vi "FlexDDS-NG_USB_Example.vi"() -> ()   [LabVIEW 2010]
uses:
  <vilib>/Utility/xml.llb/Read From XML File(string).vi
  <vilib>/Utility/xml.llb/Write to XML File(string).vi
panel:
  in  "Interactive on/off":T1(ring)
  out "return count":u32=6435
  in  "Store data":enum32{"Save settings", "Don't save settings"}(tab)=enum."Don't save settings"
  in  "XML File Path WRITE":path=path "U:/Dokumente/Bachelorarbeit/Labview/FlexDDS-NG/conf/settings_s_curve_up_down.xml"
  in  "Data source":T2(tab)=enum."Generate data with function"
  in  "XML File Path READ":path=path "U:/Dokumente/Bachelorarbeit/Labview/FlexDDS-NG/conf/settings_4consecutive_falling.xml"
  in  "Select curve form":enum32{"S curve", "Exp curve"}(tab)
  in  "s curve parameters":cluster{"k":dbl}={"k"=10.0}
  in  "exp curve parameters":cluster{"k":dbl}={"k"=5.0}
  in  "parameters non-constant channel":T3={"Number of steps"=40, "time [ms]"=10000.0, "start frequency [Hz]"=80000000.0, "end frequency [Hz]"=82000000.0}
  in  "constant frequency":dbl=80000000.0 format="%#_13g"
  in  "Constant Channel":T4(ring)
  in  "CFR2 bits":T5={"Enable ASF from STP (F)"=FALSE, "Digital ramp enable (F)"=TRUE, "Digital ramp no-dwell high (F)"=FALSE, "Digital ramp no-dwell low (F)"=FALSE, "Matched latency enable (T)"=TRUE, "Parallel data port enable (F)"=FALSE}
  in  "CFR1 bits":T6={"RAM enable (F)"=FALSE, "Manual OSK external control (F)"=FALSE, "Inverse sinc filter enable (T)"=TRUE, "DDS sine (/cosine) output (F)"=FALSE, "Load LRR at I/O update (F)"=FALSE, "Autoclear digital ramp accumulator (F)"=TRUE, "Autoclear phase accumulator (F)"=FALSE, "Clear digital ramp accumulator (F)"=FALSE, "Clear phase accumulator (F)"=FALSE, "Load ARR at I/O update (F)"=FALSE, "OSK enable (F)"=FALSE, "Select Auto OSK (F)"=FALSE}
  in  "Trigger before sequence of sweeps":T7(ring)
  out "appended instruction string 2":string="dds reset\rdcp spi:CFR1=0x404000\rdcp spi:CFR2=0x80080\rdcp 0 spi:STP0=0x3FFF0000028F5C29\rdcp 1 spi:STP0=0x3FFF0000028F5C29\rdcp 0 spi:DRL=0x147C0118147BC1DB\rdcp 0 spi:DRSS=0xFFFFFFFF00000003\rdcp 0 spi:DRR=0x2D3E\rdcp 0 update:u-d\rdcp 0 update:+d\rdcp 1 spi:DRL=0x147AE148147AE148\rdcp 1 spi:DRSS=0xFFFFFFFF00000000\rdcp 1 spi:DRR=0xFFFF\rdcp 1 update:u-d\rdcp 1 update:+d\rdcp wait:1h:\rdcp wait::DROVER\rdcp 0 spi:DRL=0x147C51F1147C0118\rdcp 0 spi:DRSS=0xFFFFFFFF00000004\rdcp 0 spi:DRR=0x2F2F\rdcp 0 update:u-d\rdcp 0 update:+d\rdcp wait:1h:\rdcp wait::DROVER\rdcp 0 spi:DRL=0x147CB92D147C51F1\rdcp 0 spi:DRSS=0xFFFFFFFF00000017\rdcp 0 spi:DRR=0xD478\rdcp 0 update:u-d\rdcp 0 update:+d\rdcp wait:1h:\rdcp wait::DROVER\rdcp 0 spi:DRL=0x147D3CCC147CB92D\rdcp 0 spi:DRSS=0xFFFFFFFF00000009\rdcp 0 spi:DRR=0x4136\rdcp 0 update:u-d\rdcp 0 update:+d\rdcp wait:1h:\rdcp wait::DROVER\rdcp 0 spi:DRL=0x147DE446147D3CCC\rdcp 0 spi:DRSS=0xFFFFFFFF0000000D\rdcp 0 spi:DRR=0x4A07\rdcp 0 update:u-d\rdcp 0 update:+d\rdcp wait:1h:\rdcp wait::DROVER\rdcp 0 spi:DRL=0x147EB8D6147DE446\rdcp 0 spi:DRSS=0xFFFFFFFF0000002B\rdcp 0 spi:DRR=0xC0EC\rdcp 0 update:u-d\rdcp 0 update:+d\rdcp wait:1h:\rdcp wait::DROVER\rdcp 0 spi:DRL=0x147FC5C3147EB8D6\rdcp 0 spi:DRSS=0xFFFFFFFF00000006\rdcp 0 spi:DRR=0x1547\rdcp 0 update:u-d\rdcp 0 update:+d\rdcp wait:1h:\rdcp wait::DROVER\rdcp 0 spi:DRL=0x148118A1147FC5C3\rdcp 0 spi:DRSS=0xFFFFFFFF0000001C\rdcp 0 spi:DRR=0x4ECD\rdcp 0 update:u-d\rdcp 0 update:+d\rdcp wait:1h:\rdcp wait::DROVER\rdcp 0 spi:DRL=0x1482C174148118A1\rdcp 0 spi:DRSS=0xFFFFFFFF00000049\rdcp 0 spi:DRR=0xA3E0\rdcp 0 update:u-d\rdcp 0 update:+d\rdcp wait:1h:\rdcp wait::DROVER\rdcp 0 spi:DRL=0x1484D2A81482C174\rdcp 0 spi:DRSS=0xFFFFFFFF00000003\rdcp 0 spi:DRR=0x568\rdcp 0 update:u-d\rdcp 0 update:+d\rdcp wait:1h:\rdcp wait::DROVER\rdcp 0 spi:DRL=0x148760AD1484D2A8\rdcp 0 spi:DRSS=0xFFFFFFFF0000008C\rdcp 0 spi:DRR=0xCC25\rdcp 0 update:u-d\rdcp 0 update:+d\rdcp wait:1h:\rdcp wait::DROVER\rdcp 0 spi:DRL=0x148A8111148760AD\rdcp 0 spi:DRSS=0xFFFFFFFF00000049\rdcp 0 spi:DRR=0x56FB\rdcp 0 update:u-d\rdcp 0 update:+d\rdcp wait:1h:\rdcp wait::DROVER\rdcp 0 spi:DRL=0x148E48EB148A8111\rdcp 0 spi:DRSS=0xFFFFFFFF00000004\rdcp 0 spi:DRR=0x3F1\rdcp 0 update:u-d\rdcp 0 update:+d\rdcp wait:1h:\rdcp wait::DROVER\rdcp 0 spi:DRL=0x1492CA77148E48EB\rdcp 0 spi:DRSS=0xFFFFFFFF000000A0\rdcp 0 spi:DRR=0x8447\rdcp 0 update:u-d\rdcp 0 update:+d\rdcp wait:1h:\rdcp wait::DROVER\rdcp 0 spi:DRL=0x149811DB1492CA77\rdcp 0 spi:DRSS=0xFFFFFFFF000000D0\rdcp 0 spi:DRR=0x92C9\rdcp 0 update:u-d\rdcp 0 update:+d\rdcp wait:1h:\rdcp wait::DROVER\rdcp 0 spi:DRL=0x149E2175149811DB\rdcp 0 spi:DRSS=0xFFFFFFFF00000100\rdcp 0 spi:DRR=0x9D59\rdcp 0 update:u-d\rdcp 0 update:+d\rdcp wait:1h:\rdcp wait::DROVER\rdcp 0 spi:DRL=0x14A4EE42149E2175\rdcp 0 spi:DRSS=0xFFFFFFFF000000C7\rdcp 0 spi:DRR=0x6D05\rdcp 0 update:u-d\rdcp 0 update:+d\rdcp wait:1h:\rdcp wait::DROVER\rdcp 0 spi:DRL=0x14AC5D7114A4EE42\rdcp 0 spi:DRSS=0xFFFFFFFF00000019\rdcp 0 spi:DRR=0xC87\rdcp 0 update:u-d\rdcp 0 update:+d\rdcp wait:1h:\rdcp wait::DROVER\rdcp 0 spi:DRL=0x14B4443314AC5D71\rdcp 0 spi:DRSS=0xFFFFFFFF00000021\rdcp 0 spi:DRR=0xF8F\rdcp 0 update:u-d\rdcp 0 update:+d\rdcp wait:1h:\rdcp wait::DROVER\rdcp 0 spi:DRL=0x14BC6A7F14B44433\rdcp 0 spi:DRSS=0xFFFFFFFF0000014D\rdcp 0 spi:DRR=0x9838\rdcp 0 update:u-d\rdcp 0 update:+d\rdcp wait:1h:\rdcp wait::DROVER\rdcp 0 spi:DRL=0x14C490CB14BC6A7F\rdcp 0 spi:DRSS=0xFFFFFFFF0000014D\rdcp 0 spi:DRR=0x9838\rdcp 0 update:u-d\rdcp 0 update:+d\rdcp wait:1h:\rdcp wait::DROVER\rdcp 0 spi:DRL=0x14CC778D14C490CB\rdcp 0 spi:DRSS=0xFFFFFFFF00000021\rdcp 0 spi:DRR=0xF8F\rdcp 0 update:u-d\rdcp 0 update:+d\rdcp wait:1h:\rdcp wait::DROVER\rdcp 0 spi:DRL=0x14D3E6BC14CC778D\rdcp 0 spi:DRSS=0xFFFFFFFF00000019\rdcp 0 spi:DRR=0xC87\rdcp 0 update:u-d\rdcp 0 update:+d\rdcp wait:1h:\rdcp wait::DROVER\rdcp 0 spi:DRL=0x14DAB38914D3E6BC\rdcp 0 spi:DRSS=0xFFFFFFFF000000C7\rdcp 0 spi:DRR=0x6D05\rdcp 0 update:u-d\rdcp 0 update:+d\rdcp wait:1h:\rdcp wait::DROVER\rdcp 0 spi:DRL=0x14E0C32314DAB389\rdcp 0 spi:DRSS=0xFFFFFFFF00000100\rdcp 0 spi:DRR=0x9D59\rdcp 0 update:u-d\rdcp 0 update:+d\rdcp wait:1h:\rdcp wait::DROVER\rdcp 0 spi:DRL=0x14E60A8714E0C323\rdcp 0 spi:DRSS=0xFFFFFFFF000000D0\rdcp 0 spi:DRR=0x92C9\rdcp 0 update:u-d\rdcp 0 update:+d\rdcp wait:1h:\rdcp wait::DROVER\rdcp 0 spi:DRL=0x14EA8C1314E60A87\rdcp 0 spi:DRSS=0xFFFFFFFF000000A0\rdcp 0 spi:DRR=0x8447\rdcp 0 update:u-d\rdcp 0 update:+d\rdcp wait:1h:\rdcp wait::DROVER\rdcp 0 spi:DRL=0x14EE53ED14EA8C13\rdcp 0 spi:DRSS=0xFFFFFFFF00000004\rdcp 0 spi:DRR=0x3F1\rdcp 0 update:u-d\rdcp 0 update:+d\rdcp wait:1h:\rdcp wait::DROVER\rdcp 0 spi:DRL=0x14F1745114EE53ED\rdcp 0 spi:DRSS=0xFFFFFFFF00000049\rdcp 0 spi:DRR=0x56FB\rdcp 0 update:u-d\rdcp 0 update:+d\rdcp wait:1h:\rdcp wait::DROVER\rdcp 0 spi:DRL=0x14F4025514F17451\rdcp 0 spi:DRSS=0xFFFFFFFF0000008C\rdcp 0 spi:DRR=0xCC25\rdcp 0 update:u-d\rdcp 0 update:+d\rdcp wait:1h:\rdcp wait::DROVER\rdcp 0 spi:DRL=0x14F6138A14F40255\rdcp 0 spi:DRSS=0xFFFFFFFF00000003\rdcp 0 spi:DRR=0x568\rdcp 0 update:u-d\rdcp 0 update:+d\rdcp wait:1h:\rdcp wait::DROVER\rdcp 0 spi:DRL=0x14F7BC5D14F6138A\rdcp 0 spi:DRSS=0xFFFFFFFF00000049\rdcp 0 spi:DRR=0xA3E0\rdcp 0 update:u-d\rdcp 0 update:+d\rdcp wait:1h:\rdcp wait::DROVER\rdcp 0 spi:DRL=0x14F90F3B14F7BC5D\rdcp 0 spi:DRSS=0xFFFFFFFF0000001C\rdcp 0 spi:DRR=0x4ECD\rdcp 0 update:u-d\rdcp 0 update:+d\rdcp wait:1h:\rdcp wait::DROVER\rdcp 0 spi:DRL=0x14FA1C2814F90F3B\rdcp 0 spi:DRSS=0xFFFFFFFF00000006\rdcp 0 spi:DRR=0x1547\rdcp 0 update:u-d\rdcp 0 update:+d\rdcp wait:1h:\rdcp wait::DROVER\rdcp 0 spi:DRL=0x14FAF0B814FA1C28\rdcp 0 spi:DRSS=0xFFFFFFFF0000002B\rdcp 0 spi:DRR=0xC0EC\rdcp 0 update:u-d\rdcp 0 update:+d\rdcp wait:1h:\rdcp wait::DROVER\rdcp 0 spi:DRL=0x14FB983214FAF0B8\rdcp 0 spi:DRSS=0xFFFFFFFF0000000D\rdcp 0 spi:DRR=0x4A07\rdcp 0 update:u-d\rdcp 0 update:+d\rdcp wait:1h:\rdcp wait::DROVER\rdcp 0 spi:DRL=0x14FC1BD114FB9832\rdcp 0 spi:DRSS=0xFFFFFFFF00000009\rdcp 0 spi:DRR=0x4136\rdcp 0 update:u-d\rdcp 0 update:+d\rdcp wait:1h:\rdcp wait::DROVER\rdcp 0 spi:DRL=0x14FC830D14FC1BD1\rdcp 0 spi:DRSS=0xFFFFFFFF00000017\rdcp 0 spi:DRR=0xD478\rdcp 0 update:u-d\rdcp 0 update:+d\rdcp wait:1h:\rdcp wait::DROVER\rdcp 0 spi:DRL=0x14FCD3E614FC830D\rdcp 0 spi:DRSS=0xFFFFFFFF00000004\rdcp 0 spi:DRR=0x2F2F\rdcp 0 update:u-d\rdcp 0 update:+d\rdcp wait:1h:\rdcp wait::DROVER\rdcp 0 spi:DRL=0x14FD132314FCD3E6\rdcp 0 spi:DRSS=0xFFFFFFFF00000003\rdcp 0 spi:DRR=0x2D3E\rdcp 0 update:u-d\rdcp 0 update:+d\rdcp wait:1h:\rdcp wait::DROVER\rdcp 0 spi:DRL=0x14FD448E14FD1323\rdcp 0 spi:DRSS=0xFFFFFFFF00000002\rdcp 0 spi:DRR=0x2699\rdcp 0 update:u-d\rdcp 0 update:+d\rdcp wait:1h:\rdcp wait::DROVER\rdcp start\r"
  out "frequency-time plot":T8(graph)=[{[{"total time[ms]"=0.0, "f1 [Hz] CH0"=80013385.70184857}, {"total time[ms]"=250.0, "f1 [Hz] CH0"=80017154.97082743}, {"total time[ms]"=250.0, "f1 [Hz] CH0"=80017154.97082743}, {"total time[ms]"=500.0, "f1 [Hz] CH0"=80021973.8852612}, {"total time[ms]"=500.0, "f1 [Hz] CH0"=80021973.8852612}, {"total time[ms]"=750.0, "f1 [Hz] CH0"=80028127.2540865}, {"total time[ms]"=750.0, "f1 [Hz] CH0"=80028127.2540865}, {"total time[ms]"=1000.0, "f1 [Hz] CH0"=80035972.41992418}, {"total time[ms]"=1000.0, "f1 [Hz] CH0"=80035972.41992418}, {"total time[ms]"=1250.0, "f1 [Hz] CH0"=80045954.73982005}, {"total time[ms]"=1250.0, "f1 [Hz] CH0"=80045954.73982005}, {"total time[ms]"=1500.0, "f1 [Hz] CH0"=80058624.46150272}, {"total time[ms]"=1500.0, "f1 [Hz] CH0"=80058624.46150272}, {"total time[ms]"=1750.0, "f1 [Hz] CH0"=80074653.77468826}, {"total time[ms]"=1750.0, "f1 [Hz] CH0"=80074653.77468826}, {"total time[ms]"=2000.0, "f1 [Hz] CH0"=80094851.74635513}, {"total time[ms]"=2000.0, "f1 [Hz] CH0"=80094851.74635513}, {"total time[ms]"=2250.0, "f1 [Hz] CH0"=80120173.30034801}, {"total time[ms]"=2250.0, "f1 [Hz] CH0"=80120173.30034801}, {"total time[ms]"=2500.0, "f1 [Hz] CH0"=80151716.36004248}, {"total time[ms]"=2500.0, "f1 [Hz] CH0"=80151716.36004248}, {"total time[ms]"=2750.0, "f1 [Hz] CH0"=80190698.92979822}, {"total time[ms]"=2750.0, "f1 [Hz] CH0"=80190698.92979822}, {"total time[ms]"=3000.0, "f1 [Hz] CH0"=80238405.84404424}, {"total time[ms]"=3000.0, "f1 [Hz] CH0"=80238405.84404424}, {"total time[ms]"=3250.0, "f1 [Hz] CH0"=80296094.39606337}, {"total time[ms]"=3250.0, "f1 [Hz] CH0"=80296094.39606337}, {"total time[ms]"=3500.0, "f1 [Hz] CH0"=80364851.04761271}, {"total time[ms]"=3500.0, "f1 [Hz] CH0"=80364851.04761271}, {"total time[ms]"=3750.0, "f1 [Hz] CH0"=80445400.27765062}, {"total time[ms]"=3750.0, "f1 [Hz] CH0"=80445400.27765062}, {"total time[ms]"=4000.0, "f1 [Hz] CH0"=80537882.84273998}, {"total time[ms]"=4000.0, "f1 [Hz] CH0"=80537882.84273998}, {"total time[ms]"=4250.0, "f1 [Hz] CH0"=80641642.60164921}, {"total time[ms]"=4250.0, "f1 [Hz] CH0"=80641642.60164921}, {"total time[ms]"=4500.0, "f1 [Hz] CH0"=80755081.3375963}, {"total time[ms]"=4500.0, "f1 [Hz] CH0"=80755081.3375963}, {"total time[ms]"=4750.0, "f1 [Hz] CH0"=80875646.9982284}, {"total time[ms]"=4750.0, "f1 [Hz] CH0"=80875646.9982284}, {"total time[ms]"=5000.0, "f1 [Hz] CH0"=81000000.0}, {"total time[ms]"=5000.0, "f1 [Hz] CH0"=81000000.0}, {"total time[ms]"=5250.0, "f1 [Hz] CH0"=81124353.0017716}, {"total time[ms]"=5250.0, "f1 [Hz] CH0"=81124353.0017716}, {"total time[ms]"=5500.0, "f1 [Hz] CH0"=81244918.6624037}, {"total time[ms]"=5500.0, "f1 [Hz] CH0"=81244918.6624037}, {"total time[ms]"=5750.0, "f1 [Hz] CH0"=81358357.39835079}, {"total time[ms]"=5750.0, "f1 [Hz] CH0"=81358357.39835079}, {"total time[ms]"=6000.0, "f1 [Hz] CH0"=81462117.15726002}, {"total time[ms]"=6000.0, "f1 [Hz] CH0"=81462117.15726002}, {"total time[ms]"=6250.0, "f1 [Hz] CH0"=81554599.72234938}, {"total time[ms]"=6250.0, "f1 [Hz] CH0"=81554599.72234938}, {"total time[ms]"=6500.0, "f1 [Hz] CH0"=81635148.95238729}, {"total time[ms]"=6500.0, "f1 [Hz] CH0"=81635148.95238729}, {"total time[ms]"=6750.0, "f1 [Hz] CH0"=81703905.60393663}, {"total time[ms]"=6750.0, "f1 [Hz] CH0"=81703905.60393663}, {"total time[ms]"=7000.0, "f1 [Hz] CH0"=81761594.15595576}, {"total time[ms]"=7000.0, "f1 [Hz] CH0"=81761594.15595576}, {"total time[ms]"=7250.0, "f1 [Hz] CH0"=81809301.07020178}, {"total time[ms]"=7250.0, "f1 [Hz] CH0"=81809301.07020178}, {"total time[ms]"=7500.0, "f1 [Hz] CH0"=81848283.63995752}, {"total time[ms]"=7500.0, "f1 [Hz] CH0"=81848283.63995752}, {"total time[ms]"=7750.0, "f1 [Hz] CH0"=81879826.69965199}, {"total time[ms]"=7750.0, "f1 [Hz] CH0"=81879826.69965199}, {"total time[ms]"=8000.0, "f1 [Hz] CH0"=81905148.25364487}, {"total time[ms]"=8000.0, "f1 [Hz] CH0"=81905148.25364487}, {"total time[ms]"=8250.0, "f1 [Hz] CH0"=81925346.22531174}, {"total time[ms]"=8250.0, "f1 [Hz] CH0"=81925346.22531174}, {"total time[ms]"=8500.0, "f1 [Hz] CH0"=81941375.53849728}, {"total time[ms]"=8500.0, "f1 [Hz] CH0"=81941375.53849728}, {"total time[ms]"=8750.0, "f1 [Hz] CH0"=81954045.26017995}, {"total time[ms]"=8750.0, "f1 [Hz] CH0"=81954045.26017995}, {"total time[ms]"=9000.0, "f1 [Hz] CH0"=81964027.58007582}, {"total time[ms]"=9000.0, "f1 [Hz] CH0"=81964027.58007582}, {"total time[ms]"=9250.0, "f1 [Hz] CH0"=81971872.7459135}, {"total time[ms]"=9250.0, "f1 [Hz] CH0"=81971872.7459135}, {"total time[ms]"=9500.0, "f1 [Hz] CH0"=81978026.1147388}, {"total time[ms]"=9500.0, "f1 [Hz] CH0"=81978026.1147388}, {"total time[ms]"=9750.0, "f1 [Hz] CH0"=81982845.02917257}, {"total time[ms]"=9750.0, "f1 [Hz] CH0"=81982845.02917257}, {"total time[ms]"=10000.0, "f1 [Hz] CH0"=81986614.29815143}, {"total time[ms]"=10000.0, "f1 [Hz] CH0"=81986614.29815143}, {"total time[ms]"=10250.0, "f1 [Hz] CH0"=81989559.74861288}]}, {[{"total time[ms]"=0.0, "f1 [Hz] CH0"=80000000.0}, {"total time[ms]"=250.0, "f1 [Hz] CH0"=80000000.0}, {"total time[ms]"=250.0, "f1 [Hz] CH0"=80000000.0}, {"total time[ms]"=500.0, "f1 [Hz] CH0"=80000000.0}, {"total time[ms]"=500.0, "f1 [Hz] CH0"=80000000.0}, {"total time[ms]"=750.0, "f1 [Hz] CH0"=80000000.0}, {"total time[ms]"=750.0, "f1 [Hz] CH0"=80000000.0}, {"total time[ms]"=1000.0, "f1 [Hz] CH0"=80000000.0}, {"total time[ms]"=1000.0, "f1 [Hz] CH0"=80000000.0}, {"total time[ms]"=1250.0, "f1 [Hz] CH0"=80000000.0}, {"total time[ms]"=1250.0, "f1 [Hz] CH0"=80000000.0}, {"total time[ms]"=1500.0, "f1 [Hz] CH0"=80000000.0}, {"total time[ms]"=1500.0, "f1 [Hz] CH0"=80000000.0}, {"total time[ms]"=1750.0, "f1 [Hz] CH0"=80000000.0}, {"total time[ms]"=1750.0, "f1 [Hz] CH0"=80000000.0}, {"total time[ms]"=2000.0, "f1 [Hz] CH0"=80000000.0}, {"total time[ms]"=2000.0, "f1 [Hz] CH0"=80000000.0}, {"total time[ms]"=2250.0, "f1 [Hz] CH0"=80000000.0}, {"total time[ms]"=2250.0, "f1 [Hz] CH0"=80000000.0}, {"total time[ms]"=2500.0, "f1 [Hz] CH0"=80000000.0}, {"total time[ms]"=2500.0, "f1 [Hz] CH0"=80000000.0}, {"total time[ms]"=2750.0, "f1 [Hz] CH0"=80000000.0}, {"total time[ms]"=2750.0, "f1 [Hz] CH0"=80000000.0}, {"total time[ms]"=3000.0, "f1 [Hz] CH0"=80000000.0}, {"total time[ms]"=3000.0, "f1 [Hz] CH0"=80000000.0}, {"total time[ms]"=3250.0, "f1 [Hz] CH0"=80000000.0}, {"total time[ms]"=3250.0, "f1 [Hz] CH0"=80000000.0}, {"total time[ms]"=3500.0, "f1 [Hz] CH0"=80000000.0}, {"total time[ms]"=3500.0, "f1 [Hz] CH0"=80000000.0}, {"total time[ms]"=3750.0, "f1 [Hz] CH0"=80000000.0}, {"total time[ms]"=3750.0, "f1 [Hz] CH0"=80000000.0}, {"total time[ms]"=4000.0, "f1 [Hz] CH0"=80000000.0}, {"total time[ms]"=4000.0, "f1 [Hz] CH0"=80000000.0}, {"total time[ms]"=4250.0, "f1 [Hz] CH0"=80000000.0}, {"total time[ms]"=4250.0, "f1 [Hz] CH0"=80000000.0}, {"total time[ms]"=4500.0, "f1 [Hz] CH0"=80000000.0}, {"total time[ms]"=4500.0, "f1 [Hz] CH0"=80000000.0}, {"total time[ms]"=4750.0, "f1 [Hz] CH0"=80000000.0}, {"total time[ms]"=4750.0, "f1 [Hz] CH0"=80000000.0}, {"total time[ms]"=5000.0, "f1 [Hz] CH0"=80000000.0}, {"total time[ms]"=5000.0, "f1 [Hz] CH0"=80000000.0}, {"total time[ms]"=5250.0, "f1 [Hz] CH0"=80000000.0}, {"total time[ms]"=5250.0, "f1 [Hz] CH0"=80000000.0}, {"total time[ms]"=5500.0, "f1 [Hz] CH0"=80000000.0}, {"total time[ms]"=5500.0, "f1 [Hz] CH0"=80000000.0}, {"total time[ms]"=5750.0, "f1 [Hz] CH0"=80000000.0}, {"total time[ms]"=5750.0, "f1 [Hz] CH0"=80000000.0}, {"total time[ms]"=6000.0, "f1 [Hz] CH0"=80000000.0}, {"total time[ms]"=6000.0, "f1 [Hz] CH0"=80000000.0}, {"total time[ms]"=6250.0, "f1 [Hz] CH0"=80000000.0}, {"total time[ms]"=6250.0, "f1 [Hz] CH0"=80000000.0}, {"total time[ms]"=6500.0, "f1 [Hz] CH0"=80000000.0}, {"total time[ms]"=6500.0, "f1 [Hz] CH0"=80000000.0}, {"total time[ms]"=6750.0, "f1 [Hz] CH0"=80000000.0}, {"total time[ms]"=6750.0, "f1 [Hz] CH0"=80000000.0}, {"total time[ms]"=7000.0, "f1 [Hz] CH0"=80000000.0}, {"total time[ms]"=7000.0, "f1 [Hz] CH0"=80000000.0}, {"total time[ms]"=7250.0, "f1 [Hz] CH0"=80000000.0}, {"total time[ms]"=7250.0, "f1 [Hz] CH0"=80000000.0}, {"total time[ms]"=7500.0, "f1 [Hz] CH0"=80000000.0}, {"total time[ms]"=7500.0, "f1 [Hz] CH0"=80000000.0}, {"total time[ms]"=7750.0, "f1 [Hz] CH0"=80000000.0}, {"total time[ms]"=7750.0, "f1 [Hz] CH0"=80000000.0}, {"total time[ms]"=8000.0, "f1 [Hz] CH0"=80000000.0}, {"total time[ms]"=8000.0, "f1 [Hz] CH0"=80000000.0}, {"total time[ms]"=8250.0, "f1 [Hz] CH0"=80000000.0}, {"total time[ms]"=8250.0, "f1 [Hz] CH0"=80000000.0}, {"total time[ms]"=8500.0, "f1 [Hz] CH0"=80000000.0}, {"total time[ms]"=8500.0, "f1 [Hz] CH0"=80000000.0}, {"total time[ms]"=8750.0, "f1 [Hz] CH0"=80000000.0}, {"total time[ms]"=8750.0, "f1 [Hz] CH0"=80000000.0}, {"total time[ms]"=9000.0, "f1 [Hz] CH0"=80000000.0}, {"total time[ms]"=9000.0, "f1 [Hz] CH0"=80000000.0}, {"total time[ms]"=9250.0, "f1 [Hz] CH0"=80000000.0}, {"total time[ms]"=9250.0, "f1 [Hz] CH0"=80000000.0}, {"total time[ms]"=9500.0, "f1 [Hz] CH0"=80000000.0}, {"total time[ms]"=9500.0, "f1 [Hz] CH0"=80000000.0}, {"total time[ms]"=9750.0, "f1 [Hz] CH0"=80000000.0}, {"total time[ms]"=9750.0, "f1 [Hz] CH0"=80000000.0}, {"total time[ms]"=10000.0, "f1 [Hz] CH0"=80000000.0}, {"total time[ms]"=10000.0, "f1 [Hz] CH0"=80000000.0}, {"total time[ms]"=10250.0, "f1 [Hz] CH0"=80000000.0}]}]
  in  "Control Elements Array":T9(array[cluster])=[{"STEP"=0, "time[ms]"=250.0, "time tolerance[us]"=0.01, "CH0"=TRUE, "rel. amplitude CH0"=1.0, "phase [°] CH0"=0.0, "f0 [Hz] CH0"=80013385.70184857, "f1 [Hz] CH0"=80017154.97082743, "CH1"=TRUE, "rel. amplitude CH1"=1.0, "phase [°] CH1"=0.0, "f0 [Hz] CH1"=80000000.0, "f1 [Hz] CH1"=80000000.0}, {"STEP"=0, "time[ms]"=250.0, "time tolerance[us]"=0.01, "CH0"=TRUE, "rel. amplitude CH0"=1.0, "phase [°] CH0"=0.0, "f0 [Hz] CH0"=80017154.97082743, "f1 [Hz] CH0"=80021973.8852612, "CH1"=FALSE, "rel. amplitude CH1"=1.0, "phase [°] CH1"=0.0, "f0 [Hz] CH1"=80000000.0, "f1 [Hz] CH1"=80000000.0}, {"STEP"=0, "time[ms]"=250.0, "time tolerance[us]"=0.01, "CH0"=TRUE, "rel. amplitude CH0"=1.0, "phase [°] CH0"=0.0, "f0 [Hz] CH0"=80021973.8852612, "f1 [Hz] CH0"=80028127.2540865, "CH1"=FALSE, "rel. amplitude CH1"=1.0, "phase [°] CH1"=0.0, "f0 [Hz] CH1"=80000000.0, "f1 [Hz] CH1"=80000000.0}, {"STEP"=0, "time[ms]"=250.0, "time tolerance[us]"=0.01, "CH0"=TRUE, "rel. amplitude CH0"=1.0, "phase [°] CH0"=0.0, "f0 [Hz] CH0"=80028127.2540865, "f1 [Hz] CH0"=80035972.41992418, "CH1"=FALSE, "rel. amplitude CH1"=1.0, "phase [°] CH1"=0.0, "f0 [Hz] CH1"=80000000.0, "f1 [Hz] CH1"=80000000.0}, {"STEP"=0, "time[ms]"=250.0, "time tolerance[us]"=0.01, "CH0"=TRUE, "rel. amplitude CH0"=1.0, "phase [°] CH0"=0.0, "f0 [Hz] CH0"=80035972.41992418, "f1 [Hz] CH0"=80045954.73982005, "CH1"=FALSE, "rel. amplitude CH1"=1.0, "phase [°] CH1"=0.0, "f0 [Hz] CH1"=80000000.0, "f1 [Hz] CH1"=80000000.0}, {"STEP"=0, "time[ms]"=250.0, "time tolerance[us]"=0.01, "CH0"=TRUE, "rel. amplitude CH0"=1.0, "phase [°] CH0"=0.0, "f0 [Hz] CH0"=80045954.73982005, "f1 [Hz] CH0"=80058624.46150272, "CH1"=FALSE, "rel. amplitude CH1"=1.0, "phase [°] CH1"=0.0, "f0 [Hz] CH1"=80000000.0, "f1 [Hz] CH1"=80000000.0}, {"STEP"=0, "time[ms]"=250.0, "time tolerance[us]"=0.01, "CH0"=TRUE, "rel. amplitude CH0"=1.0, "phase [°] CH0"=0.0, "f0 [Hz] CH0"=80058624.46150272, "f1 [Hz] CH0"=80074653.77468826, "CH1"=FALSE, "rel. amplitude CH1"=1.0, "phase [°] CH1"=0.0, "f0 [Hz] CH1"=80000000.0, "f1 [Hz] CH1"=80000000.0}, {"STEP"=0, "time[ms]"=250.0, "time tolerance[us]"=0.01, "CH0"=TRUE, "rel. amplitude CH0"=1.0, "phase [°] CH0"=0.0, "f0 [Hz] CH0"=80074653.77468826, "f1 [Hz] CH0"=80094851.74635513, "CH1"=FALSE, "rel. amplitude CH1"=1.0, "phase [°] CH1"=0.0, "f0 [Hz] CH1"=80000000.0, "f1 [Hz] CH1"=80000000.0}, {"STEP"=0, "time[ms]"=250.0, "time tolerance[us]"=0.01, "CH0"=TRUE, "rel. amplitude CH0"=1.0, "phase [°] CH0"=0.0, "f0 [Hz] CH0"=80094851.74635513, "f1 [Hz] CH0"=80120173.30034801, "CH1"=FALSE, "rel. amplitude CH1"=1.0, "phase [°] CH1"=0.0, "f0 [Hz] CH1"=80000000.0, "f1 [Hz] CH1"=80000000.0}, {"STEP"=0, "time[ms]"=250.0, "time tolerance[us]"=0.01, "CH0"=TRUE, "rel. amplitude CH0"=1.0, "phase [°] CH0"=0.0, "f0 [Hz] CH0"=80120173.30034801, "f1 [Hz] CH0"=80151716.36004248, "CH1"=FALSE, "rel. amplitude CH1"=1.0, "phase [°] CH1"=0.0, "f0 [Hz] CH1"=80000000.0, "f1 [Hz] CH1"=80000000.0}, {"STEP"=0, "time[ms]"=250.0, "time tolerance[us]"=0.01, "CH0"=TRUE, "rel. amplitude CH0"=1.0, "phase [°] CH0"=0.0, "f0 [Hz] CH0"=80151716.36004248, "f1 [Hz] CH0"=80190698.92979822, "CH1"=FALSE, "rel. amplitude CH1"=1.0, "phase [°] CH1"=0.0, "f0 [Hz] CH1"=80000000.0, "f1 [Hz] CH1"=80000000.0}, {"STEP"=0, "time[ms]"=250.0, "time tolerance[us]"=0.01, "CH0"=TRUE, "rel. amplitude CH0"=1.0, "phase [°] CH0"=0.0, "f0 [Hz] CH0"=80190698.92979822, "f1 [Hz] CH0"=80238405.84404424, "CH1"=FALSE, "rel. amplitude CH1"=1.0, "phase [°] CH1"=0.0, "f0 [Hz] CH1"=80000000.0, "f1 [Hz] CH1"=80000000.0}, {"STEP"=0, "time[ms]"=250.0, "time tolerance[us]"=0.01, "CH0"=TRUE, "rel. amplitude CH0"=1.0, "phase [°] CH0"=0.0, "f0 [Hz] CH0"=80238405.84404424, "f1 [Hz] CH0"=80296094.39606337, "CH1"=FALSE, "rel. amplitude CH1"=1.0, "phase [°] CH1"=0.0, "f0 [Hz] CH1"=80000000.0, "f1 [Hz] CH1"=80000000.0}, {"STEP"=0, "time[ms]"=250.0, "time tolerance[us]"=0.01, "CH0"=TRUE, "rel. amplitude CH0"=1.0, "phase [°] CH0"=0.0, "f0 [Hz] CH0"=80296094.39606337, "f1 [Hz] CH0"=80364851.04761271, "CH1"=FALSE, "rel. amplitude CH1"=1.0, "phase [°] CH1"=0.0, "f0 [Hz] CH1"=80000000.0, "f1 [Hz] CH1"=80000000.0}, {"STEP"=0, "time[ms]"=250.0, "time tolerance[us]"=0.01, "CH0"=TRUE, "rel. amplitude CH0"=1.0, "phase [°] CH0"=0.0, "f0 [Hz] CH0"=80364851.04761271, "f1 [Hz] CH0"=80445400.27765062, "CH1"=FALSE, "rel. amplitude CH1"=1.0, "phase [°] CH1"=0.0, "f0 [Hz] CH1"=80000000.0, "f1 [Hz] CH1"=80000000.0}, {"STEP"=0, "time[ms]"=250.0, "time tolerance[us]"=0.01, "CH0"=TRUE, "rel. amplitude CH0"=1.0, "phase [°] CH0"=0.0, "f0 [Hz] CH0"=80445400.27765062, "f1 [Hz] CH0"=80537882.84273998, "CH1"=FALSE, "rel. amplitude CH1"=1.0, "phase [°] CH1"=0.0, "f0 [Hz] CH1"=80000000.0, "f1 [Hz] CH1"=80000000.0}, {"STEP"=0, "time[ms]"=250.0, "time tolerance[us]"=0.01, "CH0"=TRUE, "rel. amplitude CH0"=1.0, "phase [°] CH0"=0.0, "f0 [Hz] CH0"=80537882.84273998, "f1 [Hz] CH0"=80641642.60164921, "CH1"=FALSE, "rel. amplitude CH1"=1.0, "phase [°] CH1"=0.0, "f0 [Hz] CH1"=80000000.0, "f1 [Hz] CH1"=80000000.0}, {"STEP"=0, "time[ms]"=250.0, "time tolerance[us]"=0.01, "CH0"=TRUE, "rel. amplitude CH0"=1.0, "phase [°] CH0"=0.0, "f0 [Hz] CH0"=80641642.60164921, "f1 [Hz] CH0"=80755081.3375963, "CH1"=FALSE, "rel. amplitude CH1"=1.0, "phase [°] CH1"=0.0, "f0 [Hz] CH1"=80000000.0, "f1 [Hz] CH1"=80000000.0}, {"STEP"=0, "time[ms]"=250.0, "time tolerance[us]"=0.01, "CH0"=TRUE, "rel. amplitude CH0"=1.0, "phase [°] CH0"=0.0, "f0 [Hz] CH0"=80755081.3375963, "f1 [Hz] CH0"=80875646.9982284, "CH1"=FALSE, "rel. amplitude CH1"=1.0, "phase [°] CH1"=0.0, "f0 [Hz] CH1"=80000000.0, "f1 [Hz] CH1"=80000000.0}, {"STEP"=0, "time[ms]"=250.0, "time tolerance[us]"=0.01, "CH0"=TRUE, "rel. amplitude CH0"=1.0, "phase [°] CH0"=0.0, "f0 [Hz] CH0"=80875646.9982284, "f1 [Hz] CH0"=81000000.0, "CH1"=FALSE, "rel. amplitude CH1"=1.0, "phase [°] CH1"=0.0, "f0 [Hz] CH1"=80000000.0, "f1 [Hz] CH1"=80000000.0}, {"STEP"=0, "time[ms]"=250.0, "time tolerance[us]"=0.01, "CH0"=TRUE, "rel. amplitude CH0"=1.0, "phase [°] CH0"=0.0, "f0 [Hz] CH0"=81000000.0, "f1 [Hz] CH0"=81124353.0017716, "CH1"=FALSE, "rel. amplitude CH1"=1.0, "phase [°] CH1"=0.0, "f0 [Hz] CH1"=80000000.0, "f1 [Hz] CH1"=80000000.0}, {"STEP"=0, "time[ms]"=250.0, "time tolerance[us]"=0.01, "CH0"=TRUE, "rel. amplitude CH0"=1.0, "phase [°] CH0"=0.0, "f0 [Hz] CH0"=81124353.0017716, "f1 [Hz] CH0"=81244918.6624037, "CH1"=FALSE, "rel. amplitude CH1"=1.0, "phase [°] CH1"=0.0, "f0 [Hz] CH1"=80000000.0, "f1 [Hz] CH1"=80000000.0}, {"STEP"=0, "time[ms]"=250.0, "time tolerance[us]"=0.01, "CH0"=TRUE, "rel. amplitude CH0"=1.0, "phase [°] CH0"=0.0, "f0 [Hz] CH0"=81244918.6624037, "f1 [Hz] CH0"=81358357.39835079, "CH1"=FALSE, "rel. amplitude CH1"=1.0, "phase [°] CH1"=0.0, "f0 [Hz] CH1"=80000000.0, "f1 [Hz] CH1"=80000000.0}, {"STEP"=0, "time[ms]"=250.0, "time tolerance[us]"=0.01, "CH0"=TRUE, "rel. amplitude CH0"=1.0, "phase [°] CH0"=0.0, "f0 [Hz] CH0"=81358357.39835079, "f1 [Hz] CH0"=81462117.15726002, "CH1"=FALSE, "rel. amplitude CH1"=1.0, "phase [°] CH1"=0.0, "f0 [Hz] CH1"=80000000.0, "f1 [Hz] CH1"=80000000.0}, {"STEP"=0, "time[ms]"=250.0, "time tolerance[us]"=0.01, "CH0"=TRUE, "rel. amplitude CH0"=1.0, "phase [°] CH0"=0.0, "f0 [Hz] CH0"=81462117.15726002, "f1 [Hz] CH0"=81554599.72234938, "CH1"=FALSE, "rel. amplitude CH1"=1.0, "phase [°] CH1"=0.0, "f0 [Hz] CH1"=80000000.0, "f1 [Hz] CH1"=80000000.0}, {"STEP"=0, "time[ms]"=250.0, "time tolerance[us]"=0.01, "CH0"=TRUE, "rel. amplitude CH0"=1.0, "phase [°] CH0"=0.0, "f0 [Hz] CH0"=81554599.72234938, "f1 [Hz] CH0"=81635148.95238729, "CH1"=FALSE, "rel. amplitude CH1"=1.0, "phase [°] CH1"=0.0, "f0 [Hz] CH1"=80000000.0, "f1 [Hz] CH1"=80000000.0}, {"STEP"=0, "time[ms]"=250.0, "time tolerance[us]"=0.01, "CH0"=TRUE, "rel. amplitude CH0"=1.0, "phase [°] CH0"=0.0, "f0 [Hz] CH0"=81635148.95238729, "f1 [Hz] CH0"=81703905.60393663, "CH1"=FALSE, "rel. amplitude CH1"=1.0, "phase [°] CH1"=0.0, "f0 [Hz] CH1"=80000000.0, "f1 [Hz] CH1"=80000000.0}, {"STEP"=0, "time[ms]"=250.0, "time tolerance[us]"=0.01, "CH0"=TRUE, "rel. amplitude CH0"=1.0, "phase [°] CH0"=0.0, "f0 [Hz] CH0"=81703905.60393663, "f1 [Hz] CH0"=81761594.15595576, "CH1"=FALSE, "rel. amplitude CH1"=1.0, "phase [°] CH1"=0.0, "f0 [Hz] CH1"=80000000.0, "f1 [Hz] CH1"=80000000.0}, {"STEP"=0, "time[ms]"=250.0, "time tolerance[us]"=0.01, "CH0"=TRUE, "rel. amplitude CH0"=1.0, "phase [°] CH0"=0.0, "f0 [Hz] CH0"=81761594.15595576, "f1 [Hz] CH0"=81809301.07020178, "CH1"=FALSE, "rel. amplitude CH1"=1.0, "phase [°] CH1"=0.0, "f0 [Hz] CH1"=80000000.0, "f1 [Hz] CH1"=80000000.0}, {"STEP"=0, "time[ms]"=250.0, "time tolerance[us]"=0.01, "CH0"=TRUE, "rel. amplitude CH0"=1.0, "phase [°] CH0"=0.0, "f0 [Hz] CH0"=81809301.07020178, "f1 [Hz] CH0"=81848283.63995752, "CH1"=FALSE, "rel. amplitude CH1"=1.0, "phase [°] CH1"=0.0, "f0 [Hz] CH1"=80000000.0, "f1 [Hz] CH1"=80000000.0}, {"STEP"=0, "time[ms]"=250.0, "time tolerance[us]"=0.01, "CH0"=TRUE, "rel. amplitude CH0"=1.0, "phase [°] CH0"=0.0, "f0 [Hz] CH0"=81848283.63995752, "f1 [Hz] CH0"=81879826.69965199, "CH1"=FALSE, "rel. amplitude CH1"=1.0, "phase [°] CH1"=0.0, "f0 [Hz] CH1"=80000000.0, "f1 [Hz] CH1"=80000000.0}, {"STEP"=0, "time[ms]"=250.0, "time tolerance[us]"=0.01, "CH0"=TRUE, "rel. amplitude CH0"=1.0, "phase [°] CH0"=0.0, "f0 [Hz] CH0"=81879826.69965199, "f1 [Hz] CH0"=81905148.25364487, "CH1"=FALSE, "rel. amplitude CH1"=1.0, "phase [°] CH1"=0.0, "f0 [Hz] CH1"=80000000.0, "f1 [Hz] CH1"=80000000.0}, {"STEP"=0, "time[ms]"=250.0, "time tolerance[us]"=0.01, "CH0"=TRUE, "rel. amplitude CH0"=1.0, "phase [°] CH0"=0.0, "f0 [Hz] CH0"=81905148.25364487, "f1 [Hz] CH0"=81925346.22531174, "CH1"=FALSE, "rel. amplitude CH1"=1.0, "phase [°] CH1"=0.0, "f0 [Hz] CH1"=80000000.0, "f1 [Hz] CH1"=80000000.0}, {"STEP"=0, "time[ms]"=250.0, "time tolerance[us]"=0.01, "CH0"=TRUE, "rel. amplitude CH0"=1.0, "phase [°] CH0"=0.0, "f0 [Hz] CH0"=81925346.22531174, "f1 [Hz] CH0"=81941375.53849728, "CH1"=FALSE, "rel. amplitude CH1"=1.0, "phase [°] CH1"=0.0, "f0 [Hz] CH1"=80000000.0, "f1 [Hz] CH1"=80000000.0}, {"STEP"=0, "time[ms]"=250.0, "time tolerance[us]"=0.01, "CH0"=TRUE, "rel. amplitude CH0"=1.0, "phase [°] CH0"=0.0, "f0 [Hz] CH0"=81941375.53849728, "f1 [Hz] CH0"=81954045.26017995, "CH1"=FALSE, "rel. amplitude CH1"=1.0, "phase [°] CH1"=0.0, "f0 [Hz] CH1"=80000000.0, "f1 [Hz] CH1"=80000000.0}, {"STEP"=0, "time[ms]"=250.0, "time tolerance[us]"=0.01, "CH0"=TRUE, "rel. amplitude CH0"=1.0, "phase [°] CH0"=0.0, "f0 [Hz] CH0"=81954045.26017995, "f1 [Hz] CH0"=81964027.58007582, "CH1"=FALSE, "rel. amplitude CH1"=1.0, "phase [°] CH1"=0.0, "f0 [Hz] CH1"=80000000.0, "f1 [Hz] CH1"=80000000.0}, {"STEP"=0, "time[ms]"=250.0, "time tolerance[us]"=0.01, "CH0"=TRUE, "rel. amplitude CH0"=1.0, "phase [°] CH0"=0.0, "f0 [Hz] CH0"=81964027.58007582, "f1 [Hz] CH0"=81971872.7459135, "CH1"=FALSE, "rel. amplitude CH1"=1.0, "phase [°] CH1"=0.0, "f0 [Hz] CH1"=80000000.0, "f1 [Hz] CH1"=80000000.0}, {"STEP"=0, "time[ms]"=250.0, "time tolerance[us]"=0.01, "CH0"=TRUE, "rel. amplitude CH0"=1.0, "phase [°] CH0"=0.0, "f0 [Hz] CH0"=81971872.7459135, "f1 [Hz] CH0"=81978026.1147388, "CH1"=FALSE, "rel. amplitude CH1"=1.0, "phase [°] CH1"=0.0, "f0 [Hz] CH1"=80000000.0, "f1 [Hz] CH1"=80000000.0}, {"STEP"=0, "time[ms]"=250.0, "time tolerance[us]"=0.01, "CH0"=TRUE, "rel. amplitude CH0"=1.0, "phase [°] CH0"=0.0, "f0 [Hz] CH0"=81978026.1147388, "f1 [Hz] CH0"=81982845.02917257, "CH1"=FALSE, "rel. amplitude CH1"=1.0, "phase [°] CH1"=0.0, "f0 [Hz] CH1"=80000000.0, "f1 [Hz] CH1"=80000000.0}, {"STEP"=0, "time[ms]"=250.0, "time tolerance[us]"=0.01, "CH0"=TRUE, "rel. amplitude CH0"=1.0, "phase [°] CH0"=0.0, "f0 [Hz] CH0"=81982845.02917257, "f1 [Hz] CH0"=81986614.29815143, "CH1"=FALSE, "rel. amplitude CH1"=1.0, "phase [°] CH1"=0.0, "f0 [Hz] CH1"=80000000.0, "f1 [Hz] CH1"=80000000.0}, {"STEP"=0, "time[ms]"=250.0, "time tolerance[us]"=0.01, "CH0"=TRUE, "rel. amplitude CH0"=1.0, "phase [°] CH0"=0.0, "f0 [Hz] CH0"=81986614.29815143, "f1 [Hz] CH0"=81989559.74861288, "CH1"=FALSE, "rel. amplitude CH1"=1.0, "phase [°] CH1"=0.0, "f0 [Hz] CH1"=80000000.0, "f1 [Hz] CH1"=80000000.0}]
  out "error out":errorcluster={"status"=TRUE, "code"=-1073807339, "source"="VISA Read in FlexDDS-NG_USB_Example.vi"}
  out "read buffer":string
  in  "FlexDDS-NG USB VISA resource name (COM)":refnum<visa-resource-name>="COM5"
  # "STEP"
  # "time [ms]"
  # "time tolerance [us]"
  # "CH0 [false=wait, keep phase&amplitude]"
  # "rel. amplitude CH0"
  # "phase [°] CH0"
  # "f0 [Hz] CH0"
  # "f1 [Hz] CH0"
  # "CH1 [false=wait, keep phase&amplitude]"
  # "rel. amplitude CH1"
  # "phase [°] CH1"
  # "f0 [Hz] CH1"
  # "f1 [Hz] CH1"
  # "f(t) = f0 + (f1-f0)/(1+exp(-k/Dt * (t-Dt/2)))"
  # "f(t) = f1 - (f1-f0)*exp(-K*t/Dt)"
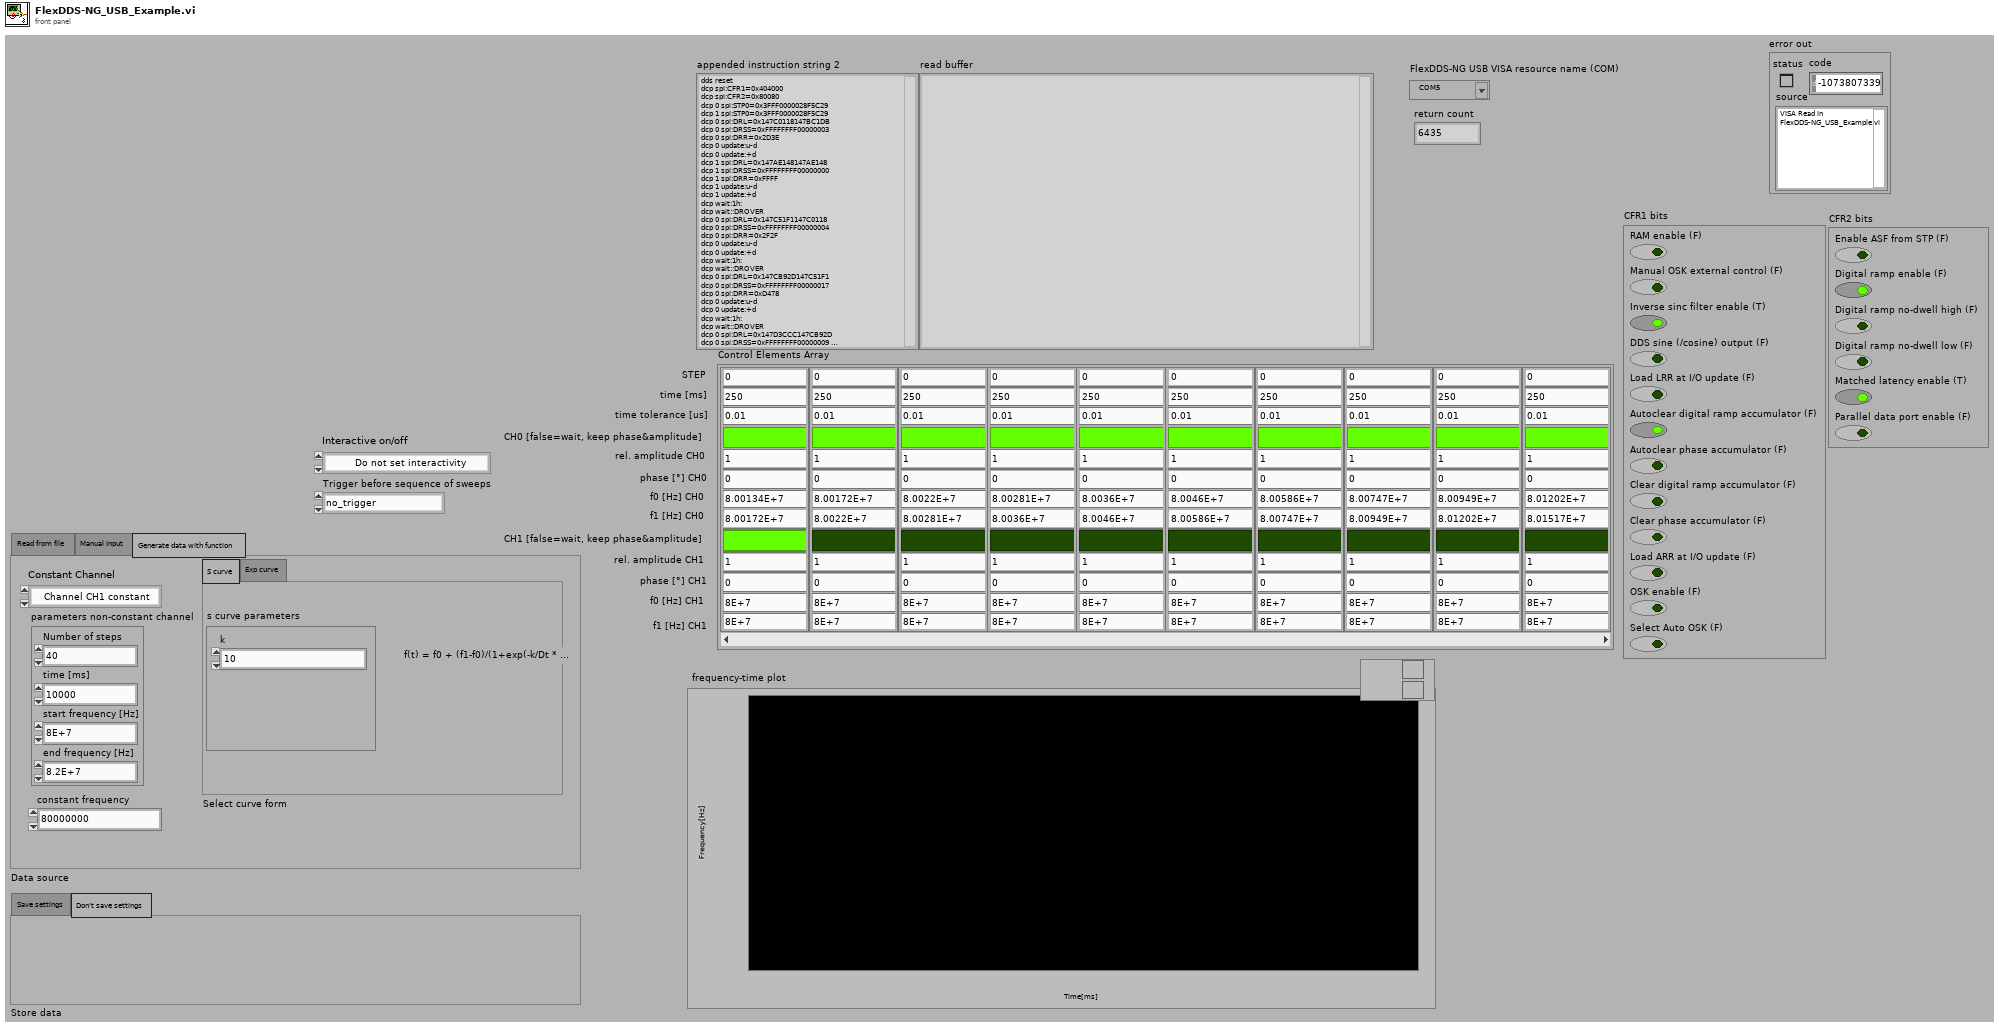
[diagram p1: front panel]
types:
  T1 = enum16{"Do not set interactivity", "Interactive off", "Interactive on"}
  T2 = enum32{"Read from file", "Manual Input", "Generate data with function"}
  T3 = cluster{"Number of steps":i32, "time [ms]":dbl, "start frequency [Hz]":dbl, "end frequency [Hz]":dbl}
  T4 = enum16{"Channel CH1 constant", "Channel CH0 constant"}
  T5 = cluster{"Enable ASF from STP (F)":bool, "Digital ramp enable (F)":bool, "Digital ramp no-dwell high (F)":bool, "Digital ramp no-dwell low (F)":bool, "Matched latency enable (T)":bool, "Parallel data port enable (F)":bool}
  T6 = cluster{"RAM enable (F)":bool, "Manual OSK external control (F)":bool, "Inverse sinc filter enable (T)":bool, "DDS sine (/cosine) output (F)":bool, "Load LRR at I/O update (F)":bool, "Autoclear digital ramp accumulator (F)":bool, "Autoclear phase accumulator (F)":bool, "Clear digital ramp accumulator (F)":bool, "Clear phase accumulator (F)":bool, "Load ARR at I/O update (F)":bool, "OSK enable (F)":bool, "Select Auto OSK (F)":bool}
  T7 = enum16{"no_trigger", "BNC_IN_A_RISING", "BNC_IN_A_FALLING", "BNC_IN_B_RISING", "BNC_IN_B_FALLING", "BNC_IN_C_RISING", "BNC_IN_C_FALLING"}
  T8 = cluster{cluster{"total time[ms]":dbl, "f1 [Hz] CH0":dbl}[]}[]
  T9 = cluster{"STEP":i32, "time[ms]":dbl, "time tolerance[us]":dbl, "CH0":bool, "rel. amplitude CH0":dbl, "phase [°] CH0":dbl, "f0 [Hz] CH0":dbl, "f1 [Hz] CH0":dbl, "CH1":bool, "rel. amplitude CH1":dbl, "phase [°] CH1":dbl, "f0 [Hz] CH1":dbl, "f1 [Hz] CH1":dbl}[]
  T10 = cluster{i32, dbl, "time tolerance":dbl, bool, dbl, dbl, "constant frequency":dbl, "constant frequency":dbl, bool, dbl, dbl, "constant frequency":dbl, "constant frequency":dbl}[]
  T11 = cluster{i32, dbl, "time tolerance":dbl, bool, dbl, dbl, "constant frequency":dbl, "constant frequency":dbl, bool, dbl, dbl, "constant frequency":dbl, "constant frequency":dbl}
  T12 = cluster{"total time[ms]":dbl, "f1 [Hz] CH1":dbl}[]
  T13 = cluster{"total time[ms]":dbl, "f1 [Hz] CH0":dbl}[]
  T14 = cluster{"STEP":i32, "time[ms]":dbl, "time tolerance[us]":dbl, "CH0":bool, "rel. amplitude CH0":dbl, "phase [°] CH0":dbl, "f0 [Hz] CH0":dbl, "f1 [Hz] CH0":dbl, "CH1":bool, "rel. amplitude CH1":dbl, "phase [°] CH1":dbl, "f0 [Hz] CH1":dbl, "f1 [Hz] CH1":dbl}
  T15 = cluster{"Array":cluster{"total time[ms]":dbl, "f1 [Hz] CH0":dbl}[]}
  T16 = cluster{"Array":cluster{"total time[ms]":dbl, "f1 [Hz] CH1":dbl}[]}
  T17 = cluster{"Array":cluster{"total time[ms]":dbl, "f1 [Hz] CH1":dbl}[]}[]
  T18 = enum32{"Channel 0", "Channel 1", "Both channels"}
  T19 = enum32{"O_RAMP_SWP_OVR", "RAM_SWP_OVR", "O_DROVER", "DROVER", "O_SPI_FIFO_EV1", "SPI_FIFO_EV1", "O_SPI_FIFO_EV0", "SPI_FIFO_EV0", "O_SPI_FIFO_FLUSHED", "SPI_FIFO_FLUSHED", "BNC_IN_B_LEVEL", "BNC_IN_B_FALLING", "BNC_IN_B_RISING", "BNC_IN_A_LEVEL", "BNC_IN_A_FALLING", "BNC_IN_A_RISING", "ALL_SPI_FIFOS_FLUSHED", "NONE"}
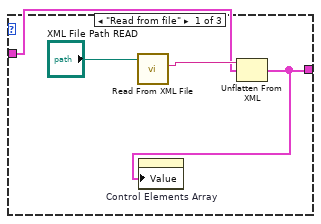
[diagram p2: hidden frame]
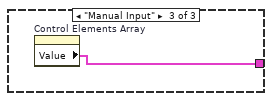
[diagram p3: hidden frame]
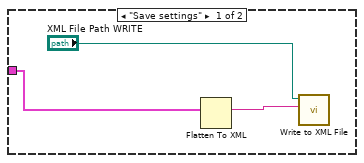
[diagram p4: hidden frame]
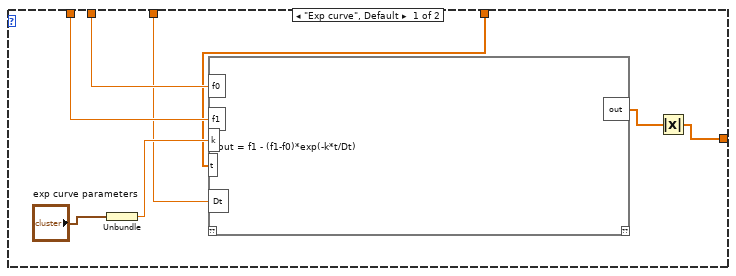
[diagram p8: hidden frame]
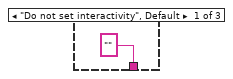
[diagram p9: hidden frame]
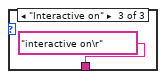
[diagram p10: hidden frame]
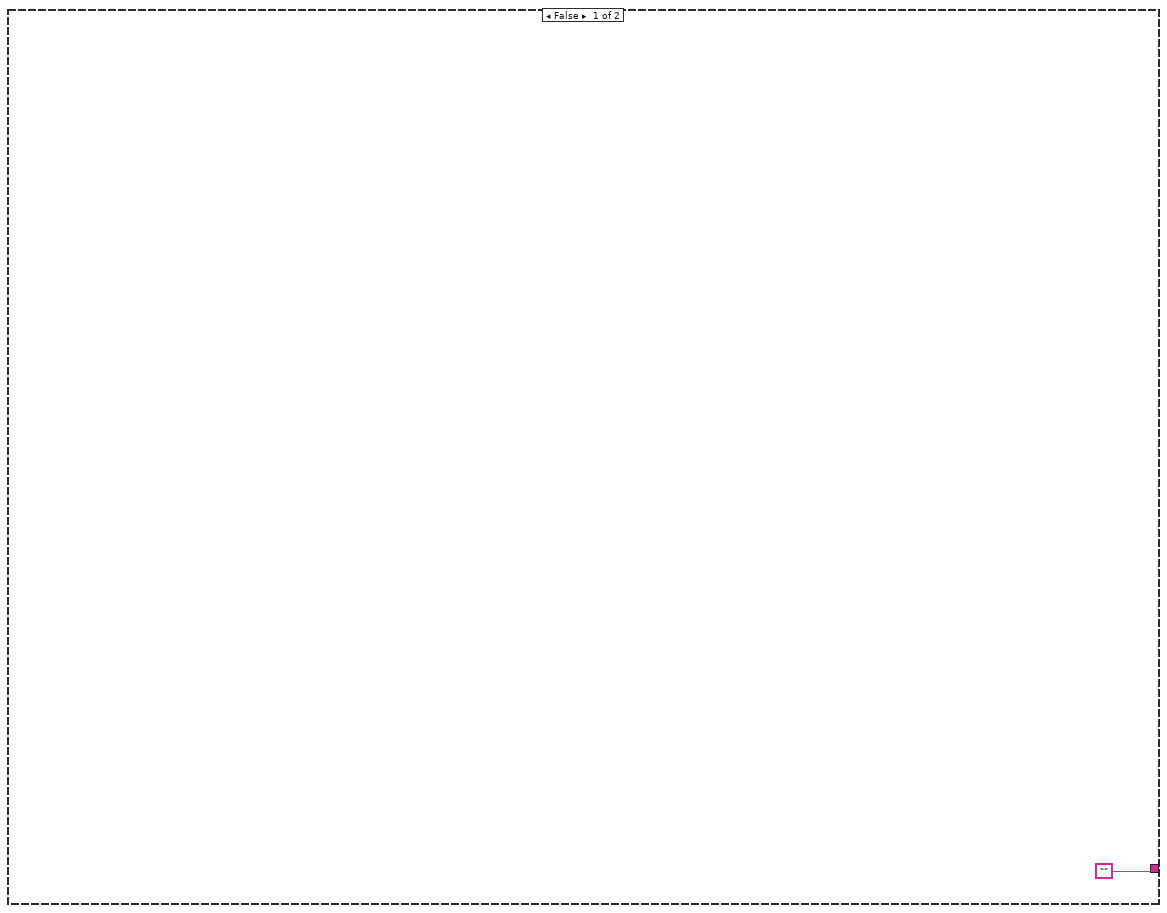
[diagram p11: hidden frame]
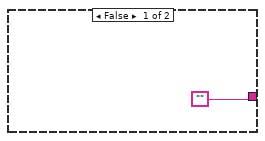
[diagram p15: hidden frame]
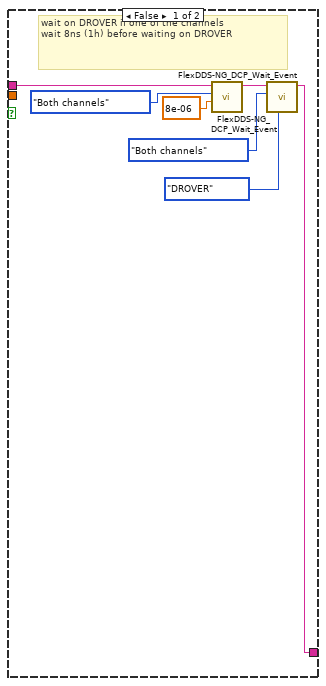
[diagram p16: hidden frame]
diagram:
  # "Relevant subvis for 'high level use':\nDCP Reset\nDCP Write STP\nDCP Write CFR1\nDCP Write CFR2\nDCP Write DRL\nDCP Write DRR\nDCP CMD (Bool)\nDCP Wait BNC\nDCP Wait Event\nDCP Start Stop\nTime To M/P\nDCP Sweep"
  n1 = stacked-sequence {
    tunnel: [w29] -> w5
    frame #0 {
      # "generate pattern from formula\nat the moment: equidistant steps\nTODO: 1. as smooth as possible (weight with 1/f'(x))"
      n2 = Unbundle("parameters non-constant channel") -> ("Number of steps"=w28:i32, "time [ms]"=w26:dbl, "start frequency [Hz]"=w25:dbl, "end frequency [Hz]"=w24:dbl)
      n3 = Increment(x=w28) -> (x+1=w30:i32)
      n4 = for {
        N: w30 -> [w59]
        tunnel: w26 -> [w47]
        tunnel: w25 -> [w56]
        tunnel: w24 -> [w57]
        shift-right: [w31] -> w29
        shift-left: T10 [] -> [w32]
        i -> [w50]
        w62 = 1.0
        w61 = 0.0
        w63 = 0.01  # time tolerance
        # "N: number of points (=number of steps+1)"
        n5 = Decrement(x=w59) -> (x-1=w58:i32)
        n6 = Increment(x=w50) -> (x+1=w49:i32)
        n7 = Build Array(w50, w49) -> (w48:i32[])
        n8 = Divide(x=w47, y=w58) -> (x/y=w54:dbl)
        n9 = Multiply(x=w54, y=w48) -> (x*y=w55:dbl[])
        n10 = case shown="\"S curve\"" "Select curve form" {
          tunnel: w57 -> [w82 w89]
          tunnel: w56 -> [w83 w90]
          tunnel: w55 -> [w77 w87]
          tunnel: w47 -> [w78 w86]
          tunnel: [w76 w84] -> w46
          frame "Exp curve", Default {
            n11 = Unbundle("exp curve parameters") -> ("k"=w79:dbl)
            n12 = mathscript code="out = f1 - (f1-f0)*exp(-k*t/Dt)"("f0"=w83, "f1"=w82, "k"=w79, "t"=w77, "Dt"=w78) -> ("out"=w81:dbl[])  [unwired: 1 in, 1 out]
            n13 = Absolute Value(x=w81) -> (abs(x)=w76:dbl[])
          }
          frame "S curve" {
            n14 = Unbundle("s curve parameters") -> ("k"=w88:dbl)
            n15 = mathscript code="out = f0+(f1-f0)*power((1+exp(-k/Dt*(t-Dt/2))),-1)"("f0"=w90, "f1"=w89, "k"=w88, "t"=w87, "Dt"=w86) -> ("out"=w85:cdb[])  [unwired: 1 in, 1 out]
            n16 = Absolute Value(x=w85) -> (abs(x)=w84:dbl[])
          }
        }
        n17 = Equal To 0?(x=w50) -> (x = 0?=w53:bool)
        n18 = Select(t=TRUE, s=w53, f=FALSE) -> (s? t:f=w41:bool)
        n19 = Index Array(array=w46) -> (element #1=w37:dbl, element #2=w36:dbl)  [unwired: 2 in]
        n20 = case shown="\"Channel CH1 constant\", Default" "Constant Channel" {
          tunnel: "constant frequency" -> [w70 w71]
          tunnel: [w70 w73] -> w43
          tunnel: [w70 w74] -> w42
          tunnel: w41 -> [w69 w72]
          tunnel: [w69 w75] -> w40
          tunnel: TRUE -> [w68 w75]
          tunnel: [w68 w72] -> w38
          tunnel: w37 -> [w67 w74]
          tunnel: w36 -> [w66 w73]
          tunnel: [w67 w71] -> w35
          tunnel: [w66 w71] -> w34
          frame "Channel CH1 constant", Default {
          }
          frame "Channel CH0 constant" {
          }
        }
        n21 = Bundle(0, w54, "time tolerance"=w63, w38, w62, w61, "constant frequency"=w35, "constant frequency"=w34, w40, w62, w61, "constant frequency"=w42, "constant frequency"=w43) -> (w65:T11)  [unwired: 1 in]
        n22 = Build Array(w65) -> (w33:T10)
        n23 = Build Array (concatenate)(w32, w33) -> (w31:T10)
      }
    }
  }
  n24 = flat-sequence {
    tunnel: w5 -> [w92]
    tunnel: [w93] -> w4
    tunnel: w4 -> [w102]
    tunnel: [w102] -> w3
    tunnel: w3 -> [w108]
    tunnel: [w108] -> w2
    frame #0 {
      # "Input: read settings from xml file\nor generate data with function\nor use manual input from array"
      n25 = case shown="\"Generate data with function\"" "Data source" {
        tunnel: w92 -> [w96 w99 _]
        tunnel: [w95 w99 w100] -> w93
        frame "Read from file" {
          n26 = call-poly <vilib>:"Read From XML File.vi"("XML File Path"="XML File Path READ") -> ("XML Elements"=w97:string)  [unwired: 8 in, 2 out]
          n27 = Unflatten From XML(xml string=w97, type=w96) -> (value=w95:T10)  [unwired: 1 in, 1 out]
          n28 = property on="Control Elements Array" class="Arr (strict)"("Value"=w95) -> ()  [unwired: 2 in, 2 out]
        }
        frame "Generate data with function" {
          n29 = property on="Control Elements Array" class="Arr (strict)"("Value"=w99) -> ()  [unwired: 2 in, 2 out]
        }
        frame "Manual Input" {
          n30 = property on="Control Elements Array" class="Arr (strict)"() -> ("Value"=w100:T9)  [unwired: 2 in, 2 out]
        }
      }
    }
    frame #1 {
      # "save array/settings or don't save anything"
      n31 = case shown="\"Don't save settings\", Default" "Store data" {
        tunnel: w102 -> [w103 _]
        frame "Save settings" {
          n32 = Flatten To XML(anything=w103) -> (xml string=w105:string)
          n33 = call-poly <vilib>:"Write to XML File.vi"("XML Input"=w105, "XML File Path"="XML File Path WRITE") -> ()  [unwired: 7 in, 3 out]
        }
        frame "Don't save settings", Default {
        }
      }
    }
    frame #2 {
      w109 = 0.0  # total time[ms]
      # "plot frequency time plot AFTER reading"
      n34 = for {
        tunnel: w108 -> [w143] mode=indexing
        shift-right: [w142] -> _
        shift-left: w109 -> [w138]
        tunnel: w108 -> [w139]
        shift-right: [w117] -> w113
        shift-left: T13 [] ("Array") -> [w118]
        shift-right: [w115] -> w114
        shift-left: T12 [] ("Array") -> [w116]
        i -> [w140]
        # "iterate through linear ramps;\nif time==0: skip;\nif CHx==false: keep frequency;"
        n35 = flat-sequence {
          tunnel: w140 -> [w153]
          tunnel: w139 -> [w154]
          tunnel: [w155] -> w127
          tunnel: [w152] -> w126
          frame #0 {
            # "i: current index\nif CHx == false, look for largest index j<i with CHx=true (to determine which frequency to plot)"
            n36 = while {
              tunnel: w153 -> [w175]
              tunnel: w154 -> [w172]
              tunnel: [w170] -> w155
              i -> [w174]
              stop <- w168 stop-if-true
              n37 = Subtract(x=w175, y=w174) -> (x-y=w173:i32)
              n38 = Index Array(array=w172, index=w173) -> (element=w171:T14)
              n39 = Unbundle By Name(w171) -> ("f1 [Hz] CH0"=w170:dbl, "CH0"=w167:bool, "time[ms]"=w169:dbl)
              n40 = Not Equal To 0?(x=w169) -> (x != 0?=w166:bool)
              n41 = And(x=w167, y=w166) -> (x .and. y?=w168:bool)
            }
            n42 = while {
              tunnel: w153 -> [w165]
              tunnel: w154 -> [w162]
              tunnel: [w160] -> w152
              i -> [w164]
              stop <- w158 stop-if-true
              n43 = Subtract(x=w165, y=w164) -> (x-y=w163:i32)
              n44 = Index Array(array=w162, index=w163) -> (element=w161:T14)
              n45 = Unbundle By Name(w161) -> ("f1 [Hz] CH1"=w160:dbl, "CH1"=w157:bool, "time[ms]"=w159:dbl)
              n46 = Not Equal To 0?(x=w159) -> (x != 0?=w156:bool)
              n47 = And(x=w157, y=w156) -> (x .and. y?=w158:bool)
            }
          }
        }
        n48 = Unbundle By Name(w143) -> ("time[ms]"=w141:dbl, "f0 [Hz] CH0"=w131:dbl, "f1 [Hz] CH0"=w130:dbl, "f0 [Hz] CH1"=w129:dbl, "f1 [Hz] CH1"=w128:dbl, "CH0"=w133:bool, "CH1"=w132:bool)
        n49 = Add(x=w138, y=w141) -> (x+y=w142:dbl)
        n50 = Not Equal To 0?(x=w141) -> (x != 0?=w119:bool)
        n51 = Select(t=w131, s=w133, f=w127) -> (s? t:f=w135:dbl)
        n52 = Select(t=w130, s=w133, f=w127) -> (s? t:f=w134:dbl)
        n53 = Select(t=w129, s=w132, f=w126) -> (s? t:f=w137:dbl)
        n54 = Select(t=w128, s=w132, f=w126) -> (s? t:f=w136:dbl)
        n55 = Bundle("total time[ms]"=w138, "f1 [Hz] CH0"=w135) -> (w125:cluster{"total time[ms]":dbl, "f1 [Hz] CH0":dbl})  [unwired: 1 in]
        n56 = Bundle(w142, "f1 [Hz] CH0"=w134) -> (w124:cluster{dbl, "f1 [Hz] CH0":dbl})  [unwired: 1 in]
        n57 = Bundle("total time[ms]"=w138, "f1 [Hz] CH1"=w137) -> (w123:cluster{"total time[ms]":dbl, "f1 [Hz] CH1":dbl})  [unwired: 1 in]
        n58 = Bundle(w142, "f1 [Hz] CH1"=w136) -> (w122:cluster{dbl, "f1 [Hz] CH1":dbl})  [unwired: 1 in]
        n59 = Build Array(w125, w124) -> (w121:T13)
        n60 = case shown="True" w119 {
          tunnel: w118 -> [w148 w150]
          tunnel: w121 -> [_ w149]
          tunnel: [w148 w151] -> w117
          frame False {
          }
          frame True {
            n61 = Build Array (concatenate)(w150, w149) -> (w151:T13)
          }
        }
        n62 = Build Array(w123, w122) -> (w120:T12)
        n63 = case shown="True" w119 {
          tunnel: w116 -> [w144 w146]
          tunnel: w120 -> [_ w145]
          tunnel: [w144 w147] -> w115
          frame False {
          }
          frame True {
            n64 = Build Array (concatenate)(w146, w145) -> (w147:T12)
          }
        }
      }
      n65 = Bundle("Array"=w113) -> (w110:T15)  [unwired: 1 in]
      n66 = Bundle("Array"=w114) -> (w111:T16)  [unwired: 1 in]
      n67 = Build Array(w110, w111) -> (→"frequency-time plot":T17)
    }
  }
  n68 = flat-sequence {
    frame #0 {
      # "This is the central data structure, work with property nodes to simplify reading and writing settings"
    }
  }
  n69 = flat-sequence {
    tunnel: [w181] -> w12
    tunnel: [w179] -> w11
    tunnel: w2 -> [w179]
    tunnel: w12 -> [w190]
    tunnel: w11 -> [w185]
    tunnel: [w188] -> w9
    tunnel: [w185] -> w7
    tunnel: w9 -> [w193]
    tunnel: [w192] -> w8
    tunnel: w7 -> [w196]
    tunnel: [w196] -> w6
    tunnel: w8 -> [w197]
    tunnel: w6 -> [w201]
    tunnel: [w199] -> w10
    tunnel: [w428] -> w13
    tunnel: w10 -> [w427]
    frame #0 {
      # "Interactive off + Full Reset"
      n70 = case shown="\"Interactive off\"" "Interactive on/off" {
        tunnel: ["" ("input 1") "interactive off\r" ("input 1") "interactive on\r" ("input 1")] -> w176
        frame "Do not set interactivity", Default {
        }
        frame "Interactive off" {
        }
        frame "Interactive on" {
        }
      }
      n71 = Format Into String(w176) -> (resulting string=w178:string)  [unwired: 3 in, 1 out]
      n72 = call "FlexDDS-NG_DCP_Reset.vi"("full reset (yes)"=TRUE, "initial instruction string"=w178) -> ("appended instruction string"=w181:string)  [unwired: 9 in]
    }
    frame #1 {
      w189 = T18."Both channels" ("Channels")
      # "* inverse sinc filter\n* digital ramp enable\n* matched latency enable"
      # "Write CFR1 and CFR2"
      n73 = call "FlexDDS-NG_DCP_WriteCFR1_C.vi"("CFR1 bits"="CFR1 bits", "Channels"=w189, "initial instruction string"=w190) -> ("appended instruction string"=w191:string)  [unwired: 8 in]
      n74 = call "FlexDDS-NG_DCP_WriteCFR2_C.vi"("CFR2 bits"="CFR2 bits", "Channels"=w189, "initial instruction string"=w191) -> ("appended instruction string"=w188:string)  [unwired: 8 in]
    }
    frame #2 {
      # "add trigger"
      n75 = call "FlexDDS-NG_DCP_Wait_BNC.vi"("Trigger"="Trigger before sequence of sweeps", "Channels"=T18."Both channels" ("Channels 2"), "appended instruction string in"=w193) -> ("appended instruction string"=w192:string)  [unwired: 8 in]
    }
    frame #3 {
      # "iterate through array of clusters and create command string\nif 1st command is decreasing ramp add very short increasing ramp before\nignore all columns with time=0ms\nTODO: write some detailed documentation what is going on below"
      n76 = Array Size(array=w201) -> (size(s)=w202:i32)
      n77 = for {
        N: w202 -> [_]
        tunnel: w201 -> [w232] mode=indexing
        tunnel: w201 -> [w218]
        tunnel: [w231] -> w200 mode=indexing
        i -> [w230]
        # "iterate through array of time steps"
        n78 = Unbundle(w232) -> ("time[ms]"=w224:dbl, "time tolerance[us]"=w223:dbl, "CH0"=w229:bool, "rel. amplitude CH0"=w222:dbl, "phase [°] CH0"=w221:dbl, "f0 [Hz] CH0"=w228:dbl, "f1 [Hz] CH0"=w227:dbl, "CH1"=w203:bool, "rel. amplitude CH1"=w220:dbl, "phase [°] CH1"=w219:dbl, "f0 [Hz] CH1"=w226:dbl, "f1 [Hz] CH1"=w225:dbl)  [unwired: 1 out]
        n79 = flat-sequence {
          tunnel: w218 -> [w280]
          tunnel: w219 -> [w244]
          tunnel: w220 -> [w245]
          tunnel: w221 -> [w248]
          tunnel: w222 -> [w249]
          tunnel: w223 -> [w281]
          tunnel: w224 -> [w235]
          tunnel: w225 -> [w242]
          tunnel: w226 -> [w243]
          tunnel: w227 -> [w246]
          tunnel: w228 -> [w247]
          tunnel: w229 -> [w253]
          tunnel: w230 -> [w240]
          tunnel: [w240] -> w217
          tunnel: [w253] -> w216
          tunnel: [w250] -> w215
          tunnel: [w247] -> w214
          tunnel: [w246] -> w213
          tunnel: [w243] -> w212
          tunnel: [w242] -> w211
          tunnel: [w235] -> w210
          tunnel: [w281] -> w209
          tunnel: [w249] -> w208
          tunnel: [w248] -> w207
          tunnel: [w245] -> w206
          tunnel: [w244] -> w205
          tunnel: [w280] -> w204
          tunnel: w203 -> [w250]
          tunnel: [w296] -> w231
          tunnel: w217 -> [w295]
          tunnel: w216 -> [w294]
          tunnel: w215 -> [w293]
          tunnel: w214 -> [w283]
          tunnel: w213 -> [w282]
          tunnel: w212 -> [w292]
          tunnel: w211 -> [w291]
          tunnel: w210 -> [w290]
          tunnel: w209 -> [w284]
          tunnel: w208 -> [w289]
          tunnel: w207 -> [w288]
          tunnel: w206 -> [w287]
          tunnel: w205 -> [w286]
          tunnel: w204 -> [w285]
          frame #0 {
            # "0<=ampl<=1\n0<=freq<=400MHz\n0<=phase=360\nChx[0] not FALSE\ntime[0] not 0"
            # "check if input is valid\nabort otherwise"
            n80 = Equal To 0?(x=w240) -> (x = 0?=w237:bool)
            n81 = Equal To 0?(x=w235) -> (x = 0?=w236:bool)
            n82 = In Range and Coerce(upper limit=360.0, x=w248, lower limit=0.0) -> (In Range?=w260:bool)  [unwired: 1 out]
            n83 = In Range and Coerce(upper limit=360.0, x=w244, lower limit=0.0) -> (In Range?=w259:bool)  [unwired: 1 out]
            n84 = And(x=w237, y=w236) -> (x .and. y?=w234:bool)
            n85 = Not(x=w234) -> (.not. x?=w233:bool)
            n86 = Select(t=w253, s=w237, f=TRUE) -> (s? t:f=w255:bool)
            n87 = Select(t=w250, s=w237, f=TRUE) -> (s? t:f=w251:bool)
            n88 = In Range and Coerce(upper limit=400000000.0, x=w247, lower limit=0.0) -> (In Range?=w264:bool)  [unwired: 1 out]
            n89 = In Range and Coerce(upper limit=400000000.0, x=w246, lower limit=0.0) -> (In Range?=w263:bool)  [unwired: 1 out]
            n90 = In Range and Coerce(upper limit=400000000.0, x=w243, lower limit=0.0) -> (In Range?=w262:bool)  [unwired: 1 out]
            n91 = In Range and Coerce(upper limit=400000000.0, x=w242, lower limit=0.0) -> (In Range?=w261:bool)  [unwired: 1 out]
            n92 = In Range and Coerce(upper limit=1.0, x=w249, lower limit=0.0) -> (In Range?=w258:bool)  [unwired: 1 out]
            n93 = In Range and Coerce(upper limit=1.0, x=w245, lower limit=0.0) -> (In Range?=w257:bool)  [unwired: 1 out]
            n94 = Compound Arithmetic op=AND(w264, w263, w262, w261, w260, w259, w258, w257, w255, w251, w233) -> (w241:bool)
            n95 = Not(x=w241) -> (.not. x?=w239:bool)
            n96 = call "Display Message to User"("Enable"=w239) -> ("OK"=w238:bool)  [unwired: 9 in, 1 out]
            n97 = Stop(stop? (T)=w238) -> ()
          }
          frame #1 {
            n98 = Not Equal?(x=0.0, y=w290) -> (x != y?=w297:bool)
            n99 = case shown="True" w297 {
              tunnel: ["" w341] -> w296
              tunnel: w295 -> [_ w307]
              tunnel: w294 -> [_ w318]
              tunnel: w293 -> [_ w310]
              tunnel: w290 -> [_ w302]
              tunnel: w292 -> [_ w309]
              tunnel: w291 -> [_ w300]
              tunnel: w289 -> [_ w322]
              tunnel: w288 -> [_ w330]
              tunnel: w287 -> [_ w329]
              tunnel: w286 -> [_ w328]
              tunnel: w285 -> [_ w308]
              tunnel: w284 -> [_ w301]
              tunnel: w283 -> [_ w315]
              tunnel: w282 -> [_ w314]
              frame False {
              }
              frame True {
                # "1st iteration and amplitude or phase changed"
                # "skip if time is zero"
                n100 = Decrement(x=w307) -> (x-1=w340:i32)
                n101 = Not(x=w318) -> (.not. x?=w343:bool)
                n102 = Not(x=w310) -> (.not. x?=w342:bool)
                n103 = And(x=w343, y=w342) -> (x .and. y?=w344:bool)
                n104 = Index Array(array=w308, index=w340) -> (element=w313:T14)
                n105 = Unbundle By Name(w313) -> ("rel. amplitude CH0"=w336:dbl, "phase [°] CH0"=w335:dbl, "rel. amplitude CH1"=w332:dbl, "phase [°] CH1"=w331:dbl)
                n106 = Unbundle By Name(w313) -> ("CH0"=w311:bool, "CH1"=w304:bool, "f1 [Hz] CH0"=w312:dbl, "f1 [Hz] CH1"=w303:dbl)
                n107 = Equal?(x=w322, y=w336) -> (x = y?=w337:bool)
                n108 = Equal?(x=w330, y=w335) -> (x = y?=w338:bool)
                n109 = Equal?(x=w332, y=w329) -> (x = y?=w334:bool)
                n110 = And(x=w337, y=w338) -> (x .and. y?=w326:bool)
                n111 = Not(x=w326) -> (.not. x?=w325:bool)
                n112 = Equal To 0?(x=w307) -> (x = 0?=w339:bool)
                n113 = Or(x=w339, y=w325) -> (x .or. y?=w319:bool)
                n114 = And(x=w318, y=w319) -> (x .and. y?=w316:bool)
                n115 = case shown="True" w316 {
                  tunnel: w322 -> [_ w415]
                  tunnel: w330 -> [_ w414]
                  tunnel: ["" w413] -> w327
                  frame False {
                  }
                  frame True {
                    # "CH0: write stp if (i==0 or ampl/phase changed) and CH0 = true"
                    n116 = call "FlexDDS-NG_DCP_WriteSTP.vi"("phase degrees (0..360)"=w414, "amplitude (0..1)"=w415, "Channels"=T18."Channel 0", "initial instruction string"="") -> ("appended instruction string"=w413:string)  [unwired: 7 in]
                  }
                }
                n117 = Equal?(x=w331, y=w328) -> (x = y?=w333:bool)
                n118 = And(x=w334, y=w333) -> (x .and. y?=w324:bool)
                n119 = Not(x=w324) -> (.not. x?=w323:bool)
                n120 = Or(x=w339, y=w323) -> (x .or. y?=w320:bool)
                n121 = And(x=w310, y=w320) -> (x .and. y?=w317:bool)
                n122 = case shown="True" w317 {
                  tunnel: [w405 w410] -> w321
                  tunnel: w329 -> [_ w408]
                  tunnel: w328 -> [_ w407]
                  tunnel: w327 -> [w405 w406]
                  frame False {
                  }
                  frame True {
                    # "CH1: write stp if (i==0 or ampl/phase changed) and CH1 = true"
                    n123 = call "FlexDDS-NG_DCP_WriteSTP.vi"("phase degrees (0..360)"=w407, "amplitude (0..1)"=w408, "Channels"=T18."Channel 1", "initial instruction string"=w406) -> ("appended instruction string"=w410:string)  [unwired: 7 in]
                  }
                }
                n124 = case shown="True" w318 {
                  tunnel: w321 -> [w375 w382]
                  tunnel: [w375 w381] -> w306
                  tunnel: w302 -> [_ w379]
                  tunnel: w301 -> [_ w378]
                  tunnel: w315 -> [_ w380]
                  tunnel: w314 -> [_ w376]
                  tunnel: w312 -> [_ w393]
                  tunnel: w311 -> [_ w388]
                  tunnel: w308 -> [_ w386]
                  tunnel: w307 -> [_ w385]
                  frame False {
                  }
                  frame True {
                    w377 = TRUE ("x")
                    # "TODO"
                    # "sweep if CH0 = true"
                    n125 = Not Equal?(x=w380, y=w393) -> (x != y?=w391:bool)
                    n126 = while {
                      tunnel: w386 -> [w404]
                      tunnel: w385 -> [w402]
                      tunnel: [w395] -> w384
                      i -> [w403]
                      stop <- w396 stop-if-true
                      # "determine last end frequency"
                      n127 = Subtract(x=w402, y=w403) -> (x-y=w401:i32)
                      n128 = Index Array(array=w404, index=w401) -> (element=w400:T14)
                      n129 = Unbundle By Name(w400) -> ("CH0"=w397:bool, "f1 [Hz] CH0"=w395:dbl, "time[ms]"=w399:dbl)
                      n130 = Not Equal To 0?(x=w399) -> (x != 0?=w398:bool)
                      n131 = And(x=w397, y=w398) -> (x .and. y?=w396:bool)
                    }
                    n132 = And(x=w388, y=w391) -> (x .and. y?=w392:bool)
                    n133 = Not(x=w388) -> (.not. x?=w389:bool)
                    n134 = Not Equal?(x=w380, y=w384) -> (x != y?=w387:bool)
                    n135 = And(x=w389, y=w387) -> (x .and. y?=w390:bool)
                    n136 = Or(x=w392, y=w390) -> (x .or. y?=w394:bool)
                    n137 = Less?(x=w376, y=w380) -> ()  [unwired: 1 out]
                    n138 = And(x=w377, y=w394) -> ()  [unwired: 1 out]
                    n139 = call "FlexDDS-NG_DCP_Sweep.vi"("f1"=w376, "jump before ramp"=w377, "f0"=w380, "sweep time tolerance (us)"=w378, "sweep time (ms)"=w379, "Channels in"=T18."Channel 0", "initial instruction string"=w382) -> ("appended instruction string out"=w381:string)  [unwired: 4 in]
                  }
                }
                n140 = case shown="True" w310 {
                  tunnel: w306 -> [w345 w351]
                  tunnel: [w345 w350] -> w305
                  tunnel: w302 -> [_ w348]
                  tunnel: w301 -> [_ w347]
                  tunnel: w309 -> [_ w349]
                  tunnel: w300 -> [_ w352]
                  tunnel: w303 -> [_ w363]
                  tunnel: w304 -> [_ w358]
                  tunnel: w308 -> [_ w356]
                  tunnel: w307 -> [_ w355]
                  frame False {
                  }
                  frame True {
                    w346 = TRUE ("x")
                    # "TODO"
                    # "sweep if CH1 = true"
                    n141 = Not Equal?(x=w349, y=w363) -> (x != y?=w361:bool)
                    n142 = while {
                      tunnel: w356 -> [w374]
                      tunnel: w355 -> [w372]
                      tunnel: [w365] -> w354
                      i -> [w373]
                      stop <- w366 stop-if-true
                      # "determine last end frequency"
                      n143 = Subtract(x=w372, y=w373) -> (x-y=w371:i32)
                      n144 = Index Array(array=w374, index=w371) -> (element=w370:T14)
                      n145 = Unbundle By Name(w370) -> ("CH1"=w367:bool, "f1 [Hz] CH1"=w365:dbl, "time[ms]"=w369:dbl)
                      n146 = Not Equal To 0?(x=w369) -> (x != 0?=w368:bool)
                      n147 = And(x=w367, y=w368) -> (x .and. y?=w366:bool)
                    }
                    n148 = And(x=w358, y=w361) -> (x .and. y?=w362:bool)
                    n149 = Not(x=w358) -> (.not. x?=w359:bool)
                    n150 = Not Equal?(x=w349, y=w354) -> (x != y?=w357:bool)
                    n151 = And(x=w359, y=w357) -> (x .and. y?=w360:bool)
                    n152 = Less?(x=w352, y=w349) -> ()  [unwired: 1 out]
                    n153 = Or(x=w362, y=w360) -> (x .or. y?=w364:bool)
                    n154 = And(x=w346, y=w364) -> ()  [unwired: 1 out]
                    n155 = call "FlexDDS-NG_DCP_Sweep.vi"("f1"=w352, "jump before ramp"=w346, "f0"=w349, "sweep time tolerance (us)"=w347, "sweep time (ms)"=w348, "Channels in"=T18."Channel 1", "initial instruction string"=w351) -> ("appended instruction string out"=w350:string)  [unwired: 4 in]
                  }
                }
                n156 = case shown="True" w344 {
                  tunnel: [w418 w426] -> w341
                  tunnel: w302 -> [_ w425]
                  tunnel: w305 -> [w417 w424]
                  frame False {
                    # "wait on DROVER if one of the channels\nwait 8ns (1h) before waiting on DROVER"
                    n157 = call "FlexDDS-NG_DCP_Wait_Event.vi"("waiting time [ms]"=8e-06, "Channels in"=T18."Both channels", "appended instruction string in"=w417) -> ("appended instruction string"=w419:string)  [unwired: 8 in]
                    n158 = call "FlexDDS-NG_DCP_Wait_Event.vi"("Event 1"=T19."DROVER", "Channels in"=T18."Both channels", "appended instruction string in"=w419) -> ("appended instruction string"=w418:string)  [unwired: 8 in]
                  }
                  frame True {
                    # "do not wait on DROVER only if CH0\nand CH1 are false"
                    n159 = call "FlexDDS-NG_DCP_Wait_Event.vi"("waiting time [ms]"=w425, "appended instruction string in"=w424) -> ("appended instruction string"=w426:string)  [unwired: 9 in]
                  }
                }
              }
            }
          }
        }
      }
      n160 = Concatenate Strings(w200) -> (w198:string)
      n161 = Format Into String(initial string=w197, w198) -> (resulting string=w199:string)  [unwired: 2 in, 1 out]
    }
    frame #4 {
      # "start"
      n162 = call "FlexDDS-NG_DCP_StartStop.vi"("initial instruction string"=w427) -> ("appended instruction string"=w428:string)  [unwired: 10 in]
    }
  }
  n163 = call "FlexDDS-NG_USB_VISA_Open.vi"("FlexDDS-NG USB VISA resource name (COM)"="FlexDDS-NG USB VISA resource name (COM)") -> ("error out"=w15:errorcluster, "FlexDDS-NG USB VISA resource name out"=w17:refnum<visa-resource-name>)  [unwired: 9 in]
  n164 = VISA Write(VISA resource name=w17, write buffer=w13, error in (no error)=w15) -> (VISA resource name out=w18:refnum<visa-resource-name>, return count=→"return count":u32, error out=w14:errorcluster)
  n165 = VISA Read(VISA resource name=w18, byte count=u32 500, error in (no error)=w14) -> (VISA resource name out=w21:refnum<visa-resource-name>, read buffer=→"read buffer":string, error out=→"error out":errorcluster)  [unwired: 1 out]
  n166 = VISA Close(VISA resource name=w21) -> ()  [unwired: 1 in, 1 out]
  "appended instruction string 2" <- w13
